vi "FTP上传通用subvi.vi"(5 "remote path":string, 6 "error in (no error)":errorcluster caption="错误输入（无错误）", 7 "local path":path, 8 "remote port (21)":u16=21 caption="远程端口(21)", 9 "password":string caption="密码", 10 "user":string="匿名" caption="用户", 11 "host":string caption="主机") -> (3 "更新进度":u8(slide) scale=0.0..100.0, 4 "error out":errorcluster caption="错误输出")   [LabVIEW 2016]
uses:
  <vilib>/FTP/ftp2.llb/FTP File Info.ctl
  <vilib>/FTP/NI_FTP.lvlib
panel:
  in  "binary (F)":bool caption="字节(F)"
  out "FTP链接结束":bool=TRUE
  out "path info":T1={"type"=enum."link", "permissions"="", "owner"="", "group"="", "size"=0, "date"="", "name"="", "link name"=""} caption="路径信息"
  in  "active (T)":bool=TRUE caption="主动(T)"
  out "file specifications":T2(array[cluster]) caption="文件规范"
  out "file errors":errorcluster[](array[cluster]) caption="文件错误"
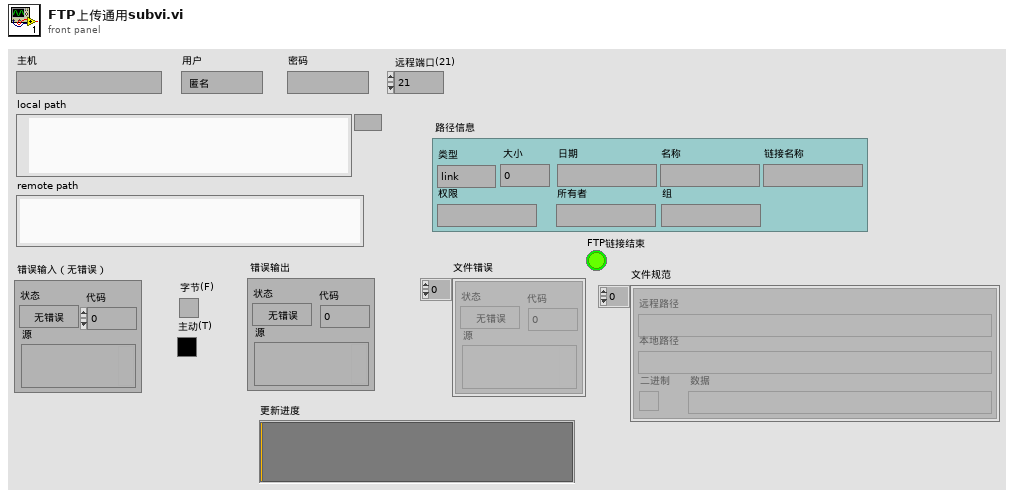
[diagram p1: front panel]
types:
  T1 = typedef "NI_FTP.lvlib/FTP File Info.ctl" = cluster{"type":enum16{"unknown", "file", "dir", "link"}, "permissions":string, "owner":string, "group":string, "size":i32, "date":string, "name":string, "link name":string}
  T2 = cluster{"remote path":string, "local path":path, "binary":bool, "data":string}[]
  T3 = cluster{"remote path":string, "local path":path, "binary":bool, "data":string}
  T4 = typedef "NI_FTP.lvlib/FTP Session.ctl" = refnum<k5>
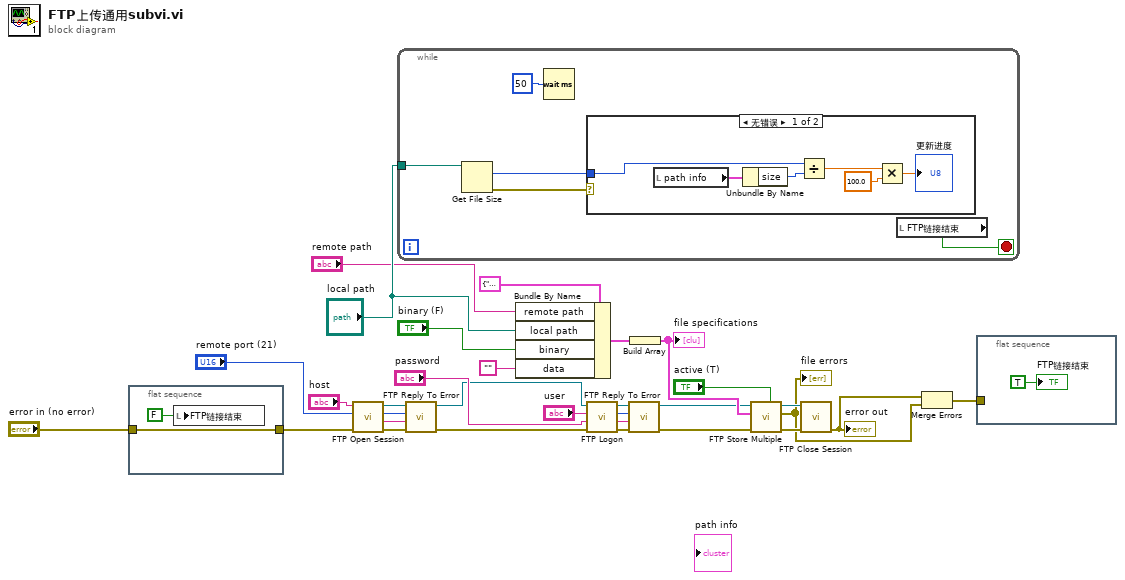
[diagram p0: block diagram]
diagram:
  n1 = flat-sequence {
    tunnel: "error in (no error)" -> [w32]
    tunnel: [w32] -> w12
    frame #0 {
      n2 = local write "FTP链接结束"(FALSE) -> ()
    }
  }
  n3 = call <vilib>:"FTP Open Session.vi"("error in (no error)"=w12, "remote port (21)"="remote port (21)", "address"="host") -> ("error out"=w29:errorcluster, "reply string"=w26:string, "reply code"=w27:i32, "ftp session"=w28:T4)  [unwired: 1 in, 4 out]
  n4 = while {
    tunnel: "local path" -> [w37]
    stop <- w34 stop-if-true
    n5 = Get File Size(file=w37) -> (size (in bytes)=w35:i64, 0:w36:errorcluster)  [unwired: 1 in, 1 out]
    n6 = Wait (ms)(milliseconds to wait=u32 50 ("等待时间（毫秒）")) -> ()  [unwired: 1 out]
    n7 = case shown="无错误" w36 {
      tunnel: w35 -> [w39 _]
      frame No Error {
        n8 = local read "path info"() -> (w44:T1)
        n9 = Unbundle By Name(w44) -> ("size"=w40:i32)
        n10 = Divide(x=w39, y=w40) -> (x/y=w43:dbl)
        n11 = Multiply(x=w43, y=100.0) -> (x*y=→"更新进度":dbl)
      }
      frame Error {
      }
    }
    n12 = local read "FTP链接结束"() -> (w34:bool)
  }
  n13 = call <vilib>:"FTP Reply To Error.vi"("error in (no error)"=w29, "reply string in"=w26, "reply code in"=w27, "ftp session"=w28) -> ("error out"=w24:errorcluster, "ftp session out"=w25:T4)  [unwired: 2 out]
  n14 = Bundle By Name(cluster=T3 {"remote path"="", "local path"=path "", "binary"=FALSE, "data"=""} ("元素"), "remote path"="remote path", "local path"="local path", "binary"="binary (F)", "data"="") -> (w10:T3)
  n15 = call <vilib>:"FTP Logon.vi"("error in (no error)"=w24, "password"="password", "user"="user", "ftp session"=w25) -> ("error out"=w23:errorcluster, "reply string"=w20:string, "reply code"=w21:i32, "ftp session out"=w22:T4)  [unwired: 4 out]
  n16 = call <vilib>:"FTP Reply To Error.vi"("error in (no error)"=w23, "reply string in"=w20, "reply code in"=w21, "ftp session"=w22) -> ("error out"=w3:errorcluster, "ftp session out"=w4:T4)  [unwired: 2 out]
  n17 = Build Array(w10) -> (w9:T2)
  "file specifications" <- w9
  n18 = call <vilib>:"FTP Store Multiple.vi"("active (T)"="active (T)", "error in (no error)"=w3, "file specifications"=w9, "ftp session"=w4) -> ("error out"=w19:errorcluster, "file errors"=w15:errorcluster[], "ftp session out"=w18:T4)  [unwired: 5 out]
  "file errors" <- w15
  n19 = call <vilib>:"FTP Close Session.vi"("error in (no error)"=w19, "ftp session"=w18) -> ("error out"=w16:errorcluster)  [unwired: 9 out]
  "error out" <- w16
  n20 = Merge Errors(w16, w15) -> (w14:errorcluster)
  n21 = flat-sequence {
    tunnel: w14 -> [_]
    frame #0 {
      "FTP链接结束" <- TRUE
    }
  }
